vi "getDir.vi"(0 "错误输入（无错误）":errorcluster) -> (1 "stripped path":path, 2 "错误输出":errorcluster)   [LabVIEW 2017]
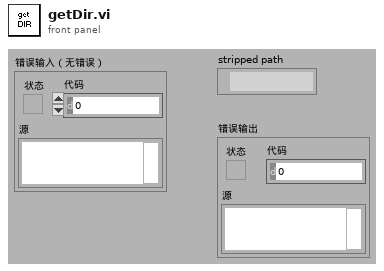
[diagram p1: front panel]
types:
  T1 = enum32{"invalid app kind", "Development System", "Run Time System", "Student Edition", "Embedded LabVIEW", "Evaluation", "Custom"}
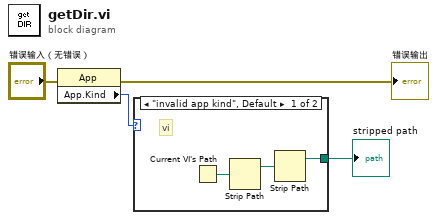
[diagram p0: block diagram]
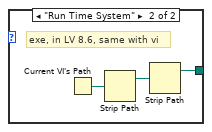
[diagram p2: hidden frame]
diagram:
  n1 = property class="App"(error in="错误输入（无错误）") -> (error out=→"错误输出":errorcluster, "App.Kind"=w1:T1)  [unwired: 1 in, 1 out]
  n2 = case shown="\"invalid app kind\", Default" w1 {
    tunnel: [w5 w8] -> w4
    frame "invalid app kind", Default {
      # "vi"
      n3 = Current VI's Path() -> (path=w7:path)
      n4 = Strip Path(path=w7) -> (stripped path=w6:path)  [unwired: 1 out]
      n5 = Strip Path(path=w6) -> (stripped path=w5:path)  [unwired: 1 out]
    }
    frame "Run Time System" {
      # "exe, in LV 8.6, same with vi"
      n6 = Current VI's Path() -> (path=w10:path)
      n7 = Strip Path(path=w10) -> (stripped path=w9:path)  [unwired: 1 out]
      n8 = Strip Path(path=w9) -> (stripped path=w8:path)  [unwired: 1 out]
    }
  }
  "stripped path" <- w4
